vi "DT_Triangle Manager_Get Oppo Point.vi"(10 "point idx 2":i32, 11 "point idx 1":i32) -> (3 "oppo point idx":i32)   [LabVIEW 2020, in "NI_AAL_Geometry.lvlib"]
uses:
  <vilib>/Analysis/NI_AAL_Geometry.lvlib
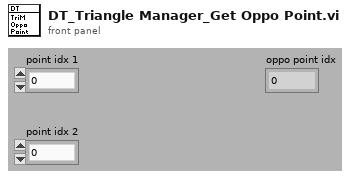
[diagram p1: front panel]
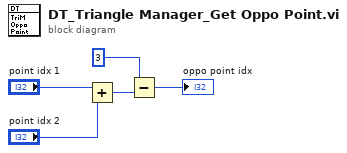
[diagram p0: block diagram]
diagram:
  n1 = Add(x="point idx 1", y="point idx 2") -> (x+y=w3:i32)
  n2 = Subtract(x=3, y=w3) -> (x-y=→"oppo point idx":i32)
